vi "3D-十字标.vi"(8 "error in (no error)":errorcluster, 9 "radius":dbl, 10 "颗粒物位置坐标":cluster{"X":dbl, "Y":dbl}[](array[cluster]) {"Y" format="%.2f"; "X" format="%.2f"}, 11 "输入图片":T1(plugin-control)) -> (0 "error out":errorcluster, 3 "输出图片":T1(plugin-control))   [LabVIEW 2017]
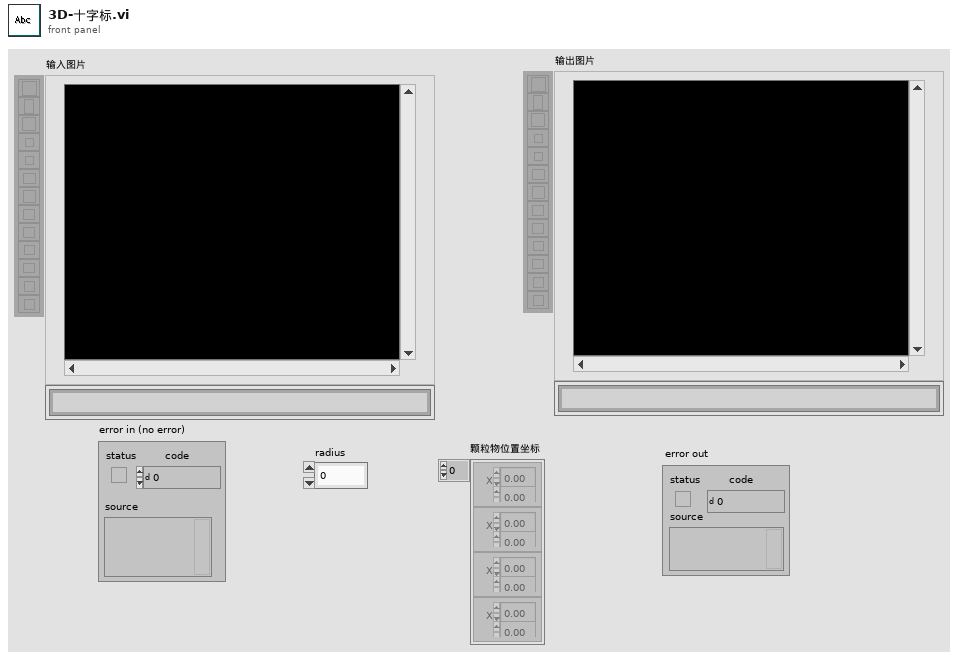
[diagram p1: front panel]
types:
  T1 = typedef "IMAQ Image.ctl" = refnum<image>
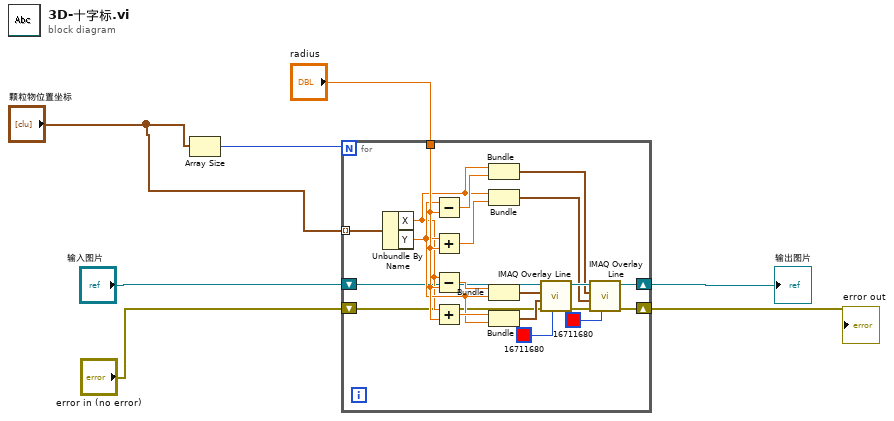
[diagram p0: block diagram]
diagram:
  n1 = Array Size(array="颗粒物位置坐标") -> (size(s)=w1:i32)
  n2 = for {
    N: w1 -> [_]
    tunnel: "radius" -> [w20]
    tunnel: "颗粒物位置坐标" -> [w8] mode=indexing
    shift-right: [w26] -> w7
    shift-left: "输入图片" -> [w10]
    shift-right: [w11] -> w5
    shift-left: "error in (no error)" -> [w9]
    n3 = Unbundle By Name(w8) -> ("X"=w16:dbl, "Y"=w19:dbl)
    n4 = Subtract(x=w19, y=w20) -> (x-y=w18:dbl)
    n5 = Add(x=w19, y=w20) -> (x+y=w17:dbl)
    n6 = Subtract(x=w16, y=w20) -> (x-y=w24:dbl)
    n7 = Add(x=w16, y=w20) -> (x+y=w23:dbl)
    n8 = Bundle("X"=w16, w18) -> (w15:cluster{"X":dbl, dbl})  [unwired: 1 in]
    n9 = Bundle("X"=w16, w17) -> (w14:cluster{"X":dbl, dbl})  [unwired: 1 in]
    n10 = Bundle(w24, "Y"=w19) -> (w22:cluster{dbl, "Y":dbl})  [unwired: 1 in]
    n11 = Bundle(w23, "Y"=w19) -> (w21:cluster{dbl, "Y":dbl})  [unwired: 1 in]
    n12 = call "IMAQ Overlay Line"("Color"=u32 16711680, "error in (no error)"=w9, "End Point"=w21, "Start Point"=w22, "Image"=w10) -> ("error out"=w25:errorcluster, "Image Out"=w27:T1)  [unwired: 5 in]
    n13 = call "IMAQ Overlay Line"("Color"=u32 16711680, "error in (no error)"=w25, "End Point"=w14, "Start Point"=w15, "Image"=w27) -> ("error out"=w11:errorcluster, "Image Out"=w26:T1)  [unwired: 5 in]
  }
  "输出图片" <- w7
  "error out" <- w5
